vi "Get.vi"(8 "error in (no error)":errorcluster, 11 "DataObject in":refnum<class "DataObject.lvclass">) -> (0 "error out":errorcluster, 3 "Conrol Value[]":T1[](array[typedef]))   [LabVIEW 2015, in "UndoLibrary.lvlib" / "DataObject.lvclass"]
uses:
  DataObject.lvclass
  Controls/cluster_Control Value.ctl
  DataObject.lvclass/DataObject.ctl
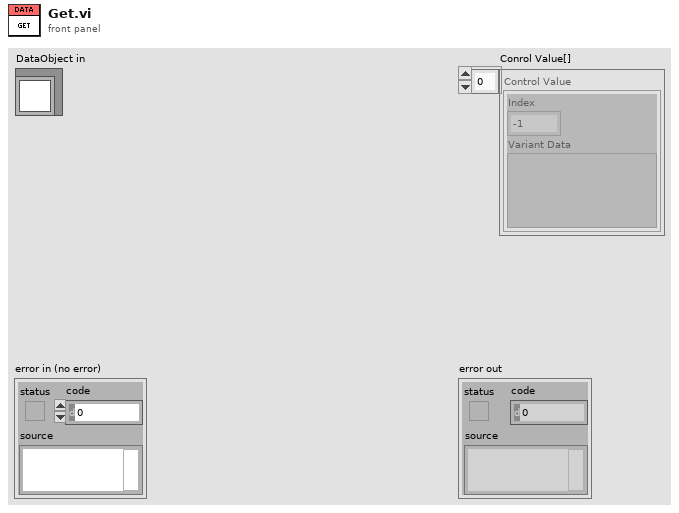
[diagram p1: front panel]
types:
  T1 = typedef "UndoLibrary.lvlib/DataObject.lvclass/cluster_Control Value.ctl" = cluster{"Index":i32, "Variant Data":variant}
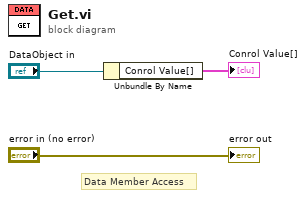
[diagram p0: block diagram]
diagram:
  # "Data Member Access"
  n1 = Unbundle By Name("DataObject in") -> ("Conrol Value[]"=→"Conrol Value[]":T1[])
  "error out" <- "error in (no error)"
